vi "OSIPI OPCUA Server.vi"(11 "Main Queue Cluster":T65) -> ()   [LabVIEW 2018]
uses:
  support/Message Queue/Message Cluster.ctl
  <vilib>/OPCUA/controls/Supported Security Policies.ctl
  Drag and Drop/State Cluster.ctl
  Drag and Drop/Thumbnail Cluster.ctl
  Drag and Drop/Object Cluster.ctl
  <vilib>/Utility/miscctls.llb/LVRectTypeDef.ctl
  Drag and Drop/Object Type Enum.ctl
  <vilib>/Utility/miscctls.llb/LVPositionTypeDef.ctl
  Config Module/Controls/Main Config Cluster.ctl
  OPC Module Config.ctl
  Scale Module Folder/Measure Instrument/State Enum.ctl
  <vilib>/Utility/miscctls.llb/LVPoint32TypeDef.ctl
  OPC Settings.ctl
  Variable Data Cluster.ctl
  <vilib>/OPCUA/controls/NodeId.ctl
  <vilib>/OPCUA/controls/OPC UA StatusCode.ctl
  <vilib>/OPCUA/controls/Subscription ID.ctl
  <vilib>/OPCUA/controls/OPC UA Client Refnum.ctl
  <vilib>/OPCUA/controls/Subscription Data Change.ctl
  <vilib>/OPCUA/controls/Data Type.ctl
  Feed Module/Controls/Feed Module Config Cluster.ctl
  Feed Module/Controls/Feed Module Settings Cluster.ctl
  Ismatec ISM 831C/Controls/Ismatech Settings Cluster.ctl
  Masterflex 7550-30/Controls/Settings Cluster.ctl
  Mettler Toledo/Controls/Settings Cluster.ctl
  Bronkhorst M13 Flow Meter/Settings Cluster.ctl
  Measure Instrument/PID 2 Parameters Cluster.ctl
  Measure Instrument/PID Input Enum.ctl
  Measure Instrument/PID 2 Output Enum.ctl
  Tacmina QI/Tacmina QI DAQ Setting.ctl
  KNF Pump/Settings Cluster plus SIMDOS.ctl
  ASIA Pump/Pump Settings.ctl
  VICI M50 Party Mode/Settings Cluster.ctl
  FLOM Pump/Settings Cluster.ctl
  SSI PR Class/SSI PR Settings Cluster.ctl
  TT Module/Controls/TT Module Config Cluster.ctl
  Acquisition/Hardware Configuration.ctl
  Acquisition/Task Cluster.ctl
  PT Module/Controls/PT Module Config Cluster.ctl
  Scale Module Folder/Feed Module/Controls/Scale Module Config Cluster.ctl
  Scale Module Folder/Feed Module/Controls/Scale Module Settings Cluster.ctl
  Pump Module Folder/Pump Module Config Cluster.ctl
  Pump Module Folder/Pump Module Settings Cluster.ctl
  LabJack Module/Controls/U3 Module Config Cluster.ctl
  Decoration Module/Decoration Module Config Cluster.ctl
  Flow Module Folder/Feed Module/Controls/Flow Module Config Cluster.ctl
  Flow Module Folder/Feed Module/Controls/Flow Module Settings Cluster.ctl
  TCU Module/TCU Module Folder/TCU Module Config Cluster.ctl
  TCU Module/TCU Module Folder/TCU Module Settings Cluster.ctl
  TCU Module/TCU Module Folder/Measure Instrument/Output Devices.ctl
  Huber TCU/Huber Settings.ctl
  Lauda Integral XT-150 TCU/Lauda Settings.ctl
  Julabo Type 1 TCU/Julabo Type 1 TCU Folder/Julabo FP-50 Settings.ctl
  Huber Unistat 410 TCU/Huber Unistat 410 Settings.ctl
  Sequencing/Squence Control.ctl
  D-O Module Folder/D-O Module Config Cluster.ctl
  D-O Module Folder/Valve Clusters.ctl
  D-O Module Folder/D-O Module Settings Cluster.ctl
  D-O Module Folder/D-O Device Settings Cluster.ctl
  VICI Electronic Actuator/VICI Electronic Actuator Settings.ctl
  Pressure Regulator Control Module/Pressure Regulator/Controls/4-20mA Module Config Cluster.ctl
  Pressure Regulator Control Module/Pressure Regulator/Controls/4-20mA Module Settings Cluster.ctl
  Pressure Transmitter/Pressure Transmitter Device Settings.ctl
  Pressure Reg Module/Pressure Regulator Device Settings.ctl
  <vilib>/OPCUA/controls/OPC UA Variable Node Refnum.ctl
  <vilib>/OPCUA/controls/OPC UA Server Refnum.ctl
  Tag VIs/Tag FGV Operation Enum.ctl
  <vilib>/OPCUA/server/Write Double.vi
  <vilib>/OPCUA/NI OPC UA Server.lvlib
  support/Message Queue/Message Queue.lvlib
  Shared Variables/Dynamic Shared Variables.lvlib
  support/Message Queue/Enqueue Message (Single).vi
  TT Module/TT Module.lvlib
  Masterflex 7550-30/Masterflex 7550-30.lvlib
  Ismatec ISM 831C/Ismatec ISM 831C.lvlib
  Tacmina QI/Tacmina QI.lvlib
  KNF Pump/KNF SIMDOS.lvlib
  VICI M50 Party Mode/VICI M6 M50 Party Mode.lvlib
  FLOM Pump/FLOM Pump.lvlib
  ASIA Pump.lvlib
  Mettler Toledo/Mettler Toledo.lvlib
  Bronkhorst M13 Flow Meter/Bronkhorst M13 Flow Meter.lvlib
  SSI PR Class/SSI PR Pump.lvlib
  Feed Module/Feed Module.lvlib
  DAQ/DAQ.lvlib
  PT Module/PT Module.lvlib
  Scale Module Folder/Scale Module.lvlib
  Pump Module Folder/Pump Module.lvlib
  LabJack Module/U3 Module.lvlib
  Flow Module Folder/Flow Module.lvlib
  Huber TCU/Huber Ministat 230 TCU.lvlib
  Lauda Integral XT-150 TCU/Lauda TCU.lvlib
  Julabo Type 1 TCU/Julabo Type 1 TCU Folder/Julabo Type FP-50 TCU.lvlib
  Huber Unistat 410 TCU/Huber Unistat 410 TCU.lvlib
  TCU Module/TCU Module Folder/TCU Module.lvlib
  Sequencing/Sequencing Library.lvlib
  D-O Module Folder/D-O Module.lvlib
  Pressure Transmitter/Pressure Transmitter Library.lvlib
  Pressure Reg Module/Pressure Regulator Library.lvlib
  Pressure Regulator Control Module/Pressure Regulator/4-20mA Module.lvlib
  OPC UA.lvlib
  Scale Module Folder/Measure Instrument/Scale Module Engine.lvlib
  Config Module/Config Module.lvlib
  Drag and Drop/Drag and Drop.lvlib
  D-O Module Folder/DIO Valve/VICI Electronic Actuator.lvlib
panel:
  out "Array 3":T3(array[cluster])
  out "OPC UA server refnum out 3":T4
  out "Array 2":T5[](array[typedef]) items=["Good"=0, "Good_SubscriptionTransferred"=2949120, "Good_CompletesAsynchronously"=3014656, "Good_Overload"=3080192, "Good_Clamped"=3145728, "Good_LocalOverride"=9830400, "Good_EntryInserted"=10616832, "Good_EntryReplaced"=10682368, "Good_NoData"=10813440, "Good_MoreData"=10878976, "Good_CommunicationEvent"=10944512, "Good_ShutdownEvent"=11010048, "Good_CallAgain"=11075584, "Good_NonCriticalTimeout"=11141120, "Good_ResultsMayBeIncomplete"=12189696, "Good_DataIgnored"=14221312, "Uncertain"=1073741824, "Uncertain_ReferenceOutOfServer"=1080819712, "Uncertain_NoCommunicationLastUsableValue"=1083113472, "Uncertain_LastUsableValue"=1083179008, "Uncertain_SubstituteValue"=1083244544, "Uncertain_InitialValue"=1083310080, "Uncertain_SensorNotAccurate"=1083375616, "Uncertain_EngineeringUnitsExceeded"=1083441152, "Uncertain_SubNormal"=1083506688, "Uncertain_DataSubNormal"=1084489728, "Uncertain_ReferenceNotDeleted"=1086062592, "Uncertain_NotAllNodesAvailable"=1086324736, "Bad"=2147483648, "Bad_UnexpectedError"=2147549184, "Bad_InternalError"=2147614720, "Bad_OutOfMemory"=2147680256, "Bad_ResourceUnavailable"=2147745792, "Bad_CommunicationError"=2147811328, "Bad_EncodingError"=2147876864, "Bad_DecodingError"=2147942400, "Bad_EncodingLimitsExceeded"=2148007936, "Bad_UnknownResponse"=2148073472, "Bad_Timeout"=2148139008, "Bad_ServiceUnsupported"=2148204544, "Bad_Shutdown"=2148270080, "Bad_ServerNotConnected"=2148335616, "Bad_ServerHalted"=2148401152, "Bad_NothingToDo"=2148466688, "Bad_TooManyOperations"=2148532224, "Bad_DataTypeIdUnknown"=2148597760, "Bad_CertificateInvalid"=2148663296, "Bad_SecurityChecksFailed"=2148728832, "Bad_CertificateTimeInvalid"=2148794368, "Bad_CertificateIssuerTimeInvalid"=2148859904, "Bad_CertificateHostNameInvalid"=2148925440, "Bad_CertificateUriInvalid"=2148990976, "Bad_CertificateUseNotAllowed"=2149056512, "Bad_CertificateIssuerUseNotAllowed"=2149122048, "Bad_CertificateUntrusted"=2149187584, "Bad_CertificateRevocationUnknown"=2149253120, "Bad_CertificateIssuerRevocationUnknown"=2149318656, "Bad_CertificateRevoked"=2149384192, "Bad_CertificateIssuerRevoked"=2149449728, "Bad_UserAccessDenied"=2149515264, "Bad_IdentityTokenInvalid"=2149580800, "Bad_IdentityTokenRejected"=2149646336, "Bad_SecureChannelIdInvalid"=2149711872, "Bad_InvalidTimestamp"=2149777408, "Bad_NonceInvalid"=2149842944, "Bad_SessionIdInvalid"=2149908480, "Bad_SessionClosed"=2149974016, "Bad_SessionNotActivated"=2150039552, "Bad_SubscriptionIdInvalid"=2150105088, "Bad_RequestHeaderInvalid"=2150236160, "Bad_TimestampsToReturnInvalid"=2150301696, "Bad_RequestCancelledByClient"=2150367232, "Bad_NoCommunication"=2150694912, "Bad_WaitingForInitialData"=2150760448, "Bad_NodeIdInvalid"=2150825984, "Bad_NodeIdUnknown"=2150891520, "Bad_AttributeIdInvalid"=2150957056, "Bad_IndexRangeInvalid"=2151022592, "Bad_IndexRangeNoData"=2151088128, "Bad_DataEncodingInvalid"=2151153664, "Bad_DataEncodingUnsupported"=2151219200, "Bad_NotReadable"=2151284736, "Bad_NotWritable"=2151350272, "Bad_OutOfRange"=2151415808, "Bad_NotSupported"=2151481344, "Bad_NotFound"=2151546880, "Bad_ObjectDeleted"=2151612416, "Bad_NotImplemented"=2151677952, "Bad_MonitoringModeInvalid"=2151743488, "Bad_MonitoredItemIdInvalid"=2151809024, "Bad_MonitoredItemFilterInvalid"=2151874560, "Bad_MonitoredItemFilterUnsupported"=2151940096, "Bad_FilterNotAllowed"=2152005632, "Bad_StructureMissing"=2152071168, "Bad_EventFilterInvalid"=2152136704, "Bad_ContentFilterInvalid"=2152202240, "Bad_FilterOperandInvalid"=2152267776, "Bad_ContinuationPointInvalid"=2152333312, "Bad_NoContinuationPoints"=2152398848, "Bad_ReferenceTypeIdInvalid"=2152464384, "Bad_BrowseDirectionInvalid"=2152529920, "Bad_NodeNotInView"=2152595456, "Bad_ServerUriInvalid"=2152660992, "Bad_ServerNameMissing"=2152726528, "Bad_DiscoveryUrlMissing"=2152792064, "Bad_SempahoreFileMissing"=2152857600, "Bad_RequestTypeInvalid"=2152923136, "Bad_SecurityModeRejected"=2152988672, "Bad_SecurityPolicyRejected"=2153054208, "Bad_TooManySessions"=2153119744, "Bad_UserSignatureInvalid"=2153185280, "Bad_ApplicationSignatureInvalid"=2153250816, "Bad_NoValidCertificates"=2153316352, "Bad_RequestCancelledByRequest"=2153381888, "Bad_ParentNodeIdInvalid"=2153447424, "Bad_ReferenceNotAllowed"=2153512960, "Bad_NodeIdRejected"=2153578496, "Bad_NodeIdExists"=2153644032, "Bad_NodeClassInvalid"=2153709568, "Bad_BrowseNameInvalid"=2153775104, "Bad_BrowseNameDuplicated"=2153840640, "Bad_NodeAttributesInvalid"=2153906176, "Bad_TypeDefinitionInvalid"=2153971712, "Bad_SourceNodeIdInvalid"=2154037248, "Bad_TargetNodeIdInvalid"=2154102784, "Bad_DuplicateReferenceNotAllowed"=2154168320, "Bad_InvalidSelfReference"=2154233856, "Bad_ReferenceLocalOnly"=2154299392, "Bad_NoDeleteRights"=2154364928, "Bad_ServerIndexInvalid"=2154430464, "Bad_ViewIdUnknown"=2154496000, "Bad_TooManyMatches"=2154627072, "Bad_QueryTooComplex"=2154692608, "Bad_NoMatch"=2154758144, "Bad_MaxAgeInvalid"=2154823680, "Bad_HistoryOperationInvalid"=2154889216, "Bad_HistoryOperationUnsupported"=2154954752, "Bad_WriteNotSupported"=2155020288, "Bad_TypeMismatch"=2155085824, "Bad_MethodInvalid"=2155151360, "Bad_ArgumentsMissing"=2155216896, "Bad_TooManySubscriptions"=2155282432, "Bad_TooManyPublishRequests"=2155347968, "Bad_NoSubscription"=2155413504, "Bad_SequenceNumberUnknown"=2155479040, "Bad_MessageNotAvailable"=2155544576, "Bad_InsufficientClientProfile"=2155610112, "Bad_TcpServerTooBusy"=2155675648, "Bad_TcpMessageTypeInvalid"=2155741184, "Bad_TcpSecureChannelUnknown"=2155806720, "Bad_TcpMessageTooLarge"=2155872256, "Bad_TcpNotEnoughResources"=2155937792, "Bad_TcpInternalError"=2156003328, "Bad_TcpEndpointUrlInvalid"=2156068864, "Bad_RequestInterrupted"=2156134400, "Bad_RequestTimeout"=2156199936, "Bad_SecureChannelClosed"=2156265472, "Bad_SecureChannelTokenUnknown"=2156331008, "Bad_SequenceNumberInvalid"=2156396544, "Bad_ConfigurationError"=2156462080, "Bad_NotConnected"=2156527616, "Bad_DeviceFailure"=2156593152, "Bad_SensorFailure"=2156658688, "Bad_OutOfService"=2156724224, "Bad_DeadbandFilterInvalid"=2156789760, "Bad_RefreshInProgress"=2157379584, "Bad_ConditionAlreadyDisabled"=2157445120, "Bad_ConditionDisabled"=2157510656, "Bad_EventIdUnknown"=2157576192, "Bad_NoData"=2157641728, "Bad_DataLost"=2157772800, "Bad_DataUnavailable"=2157838336, "Bad_EntryExists"=2157903872, "Bad_NoEntryExists"=2157969408, "Bad_TimestampNotSupported"=2158034944, "Bad_InvalidArgument"=2158690304, "Bad_ConnectionRejected"=2158755840, "Bad_Disconnect"=2158821376, "Bad_ConnectionClosed"=2158886912, "Bad_InvalidState"=2158952448, "Bad_EndOfStream"=2159017984, "Bad_NoDataAvailable"=2159083520, "Bad_WaitingForResponse"=2159149056, "Bad_OperationAbandoned"=2159214592, "Bad_ExpectedStreamToBlock"=2159280128, "Bad_WouldBlock"=2159345664, "Bad_SyntaxError"=2159411200, "Bad_MaxConnectionsReached"=2159476736, "Bad_RequestTooLarge"=2159542272, "Bad_ResponseTooLarge"=2159607808, "Bad_EventNotAcknowledgeable"=2159738880, "Bad_InvalidTimestampArgument"=2159869952, "Bad_ProtocolVersionUnsupported"=2159935488, "Bad_StateNotActive"=2160001024, "Bad_FilterOperatorInvalid"=2160132096, "Bad_FilterOperatorUnsupported"=2160197632, "Bad_FilterOperandCountMismatch"=2160263168, "Bad_FilterElementInvalid"=2160328704, "Bad_FilterLiteralInvalid"=2160394240, "Bad_IdentityChangeNotSupported"=2160459776, "Bad_NotTypeDefinition"=2160590848, "Bad_ViewTimestampInvalid"=2160656384, "Bad_ViewParameterMismatch"=2160721920, "Bad_ViewVersionInvalid"=2160787456, "Bad_ConditionAlreadyEnabled"=2160852992, "Bad_DialogNotActive"=2160918528, "Bad_DialogResponseInvalid"=2160984064, "Bad_ConditionBranchAlreadyAcked"=2161049600, "Bad_ConditionBranchAlreadyConfirmed"=2161115136, "Bad_ConditionAlreadyShelved"=2161180672, "Bad_ConditionNotShelved"=2161246208, "Bad_ShelvingTimeOutOfRange"=2161311744, "Bad_AggregateListMismatch"=2161377280, "Bad_AggregateNotSupported"=2161442816, "Bad_AggregateInvalidInputs"=2161508352, "Bad_BoundNotFound"=2161573888, "Bad_BoundNotSupported"=2161639424, "Bad_AggregateConfigurationRejected"=2161770496, "Bad_TooManyMonitoredItems"=2161836032]
  out "OPC UA server refnum out":T4
  out "Array":T3(array[cluster])
  in  "?":T6={"VI refs"=[], "Queues"=[], "[Thumbnails]"=[], "Drag Object Idx"=0, "[Objects]"=[], "Active Object"=0, "Drop Offset"={"Left"=0, "Top"=0}, "Process Name"="", "Main Config"={"OPC Module Configs"=[], "Feed Module Configs"=[], "Log File Path"=path "", "TT Module Configs"=[], "DAQ Config"={"Tasks"=[]}, "PT Module Configs"=[], "Scale Module Configs"=[], "Pump Module Configs"=[], "U3 Module Configs"=[{"GUID"="", "Drop Coords"={"Horizontal"=0, "Vertical"=0}, "AI Channel Number"=enum."Default", "Process Name"="", "Input Channel Numeric Alarm Settings"=[]}], "Decoration Module Configs"=[], "Flow Module Configs"=[], "TCU Module Configs"=[], "Steps"=[], "DO Module Configs"=[], "PR Module Configs"=[], "Cycle Period"=0.0}, "Campaign Filepath"=path "", "Config Changed?"=FALSE} {"Main Config"."PR Module Configs"."Settings"."PID 2 Parameters"."output range"."output low" format="%.2f"; "Main Config"."PR Module Configs"."Settings"."PID 2 Parameters"."output range"."output high" min=0.0 max=100.0 format="%.2f"; "Main Config"."PR Module Configs"."Settings"."PID 2 Parameters"."PID gains"."derivative time (Td, min)" format="%.3f"; "Main Config"."PR Module Configs"."Settings"."PID 2 Parameters"."PID gains"."integral time (Ti, min)" format="%.3f"; "Main Config"."PR Module Configs"."Settings"."PID 2 Parameters"."PID gains"."proportional gain (Kc)" format="%.3f"; "Main Config"."Steps"."Control" items=["Pump %", "Setpoint"]; "Main Config"."TCU Module Configs"."Settings"."Julabo FP-50 Settings"."Pump Power" min=0 max=8 step=1; "Main Config"."TCU Module Configs"."Settings"."Lauda Settings"."Pump Power" min=0 max=8 step=1; "Main Config"."Pump Module Configs"."Settings"."ASIA Pump C"."channel" min=0 max=1 step=1; "Main Config"."Pump Module Configs"."Settings"."Masterflex"."Pump Number" min=1.0 max=20.0 step=1.0; "Main Config"."Pump Module Configs"."Settings"."Ismatech"."Pump Number" min=1.0 max=20.0 step=1.0; "Main Config"."Feed Module Configs"."Settings"."output range"."output low" min=0.0 max=100.0 format="%.2f"; "Main Config"."Feed Module Configs"."Settings"."output range"."output high" format="%.2f"; "Main Config"."Feed Module Configs"."Settings"."PID 2 Parameters"."PID gains"."derivative time (Td, min)" format="%.3f"; "Main Config"."Feed Module Configs"."Settings"."PID 2 Parameters"."PID gains"."integral time (Ti, min)" format="%.3f"; "Main Config"."Feed Module Configs"."Settings"."PID 2 Parameters"."PID gains"."proportional gain (Kc)" format="%.3f"; "Main Config"."Feed Module Configs"."Settings"."ASIA Pump C"."channel" min=0 max=1 step=1; "Main Config"."Feed Module Configs"."Settings"."Ismatech"."Pump Number" min=1.0 max=20.0 step=1.0; "Main Config"."Feed Module Configs"."Settings"."Masterflex"."Pump Number" min=1.0 max=20.0 step=1.0}
  out "Tag Values":dbl[](array[numeric])
  out "Tag Names":string[](array[string])
  in  "?":T6 {"Main Config"."PR Module Configs"."Settings"."PID 2 Parameters"."output range"."output low" format="%.2f"; "Main Config"."PR Module Configs"."Settings"."PID 2 Parameters"."output range"."output high" min=0.0 max=100.0 format="%.2f"; "Main Config"."PR Module Configs"."Settings"."PID 2 Parameters"."PID gains"."derivative time (Td, min)" format="%.3f"; "Main Config"."PR Module Configs"."Settings"."PID 2 Parameters"."PID gains"."integral time (Ti, min)" format="%.3f"; "Main Config"."PR Module Configs"."Settings"."PID 2 Parameters"."PID gains"."proportional gain (Kc)" format="%.3f"; "Main Config"."Steps"."Control" items=["Pump %", "Setpoint"]; "Main Config"."TCU Module Configs"."Settings"."Julabo FP-50 Settings"."Pump Power" min=0 max=8 step=1; "Main Config"."TCU Module Configs"."Settings"."Lauda Settings"."Pump Power" min=0 max=8 step=1; "Main Config"."Pump Module Configs"."Settings"."ASIA Pump C"."channel" min=0 max=1 step=1; "Main Config"."Pump Module Configs"."Settings"."Masterflex"."Pump Number" min=1.0 max=20.0 step=1.0; "Main Config"."Pump Module Configs"."Settings"."Ismatech"."Pump Number" min=1.0 max=20.0 step=1.0; "Main Config"."Feed Module Configs"."Settings"."output range"."output low" min=0.0 max=100.0 format="%.2f"; "Main Config"."Feed Module Configs"."Settings"."output range"."output high" format="%.2f"; "Main Config"."Feed Module Configs"."Settings"."PID 2 Parameters"."PID gains"."derivative time (Td, min)" format="%.3f"; "Main Config"."Feed Module Configs"."Settings"."PID 2 Parameters"."PID gains"."integral time (Ti, min)" format="%.3f"; "Main Config"."Feed Module Configs"."Settings"."PID 2 Parameters"."PID gains"."proportional gain (Kc)" format="%.3f"; "Main Config"."Feed Module Configs"."Settings"."ASIA Pump C"."channel" min=0 max=1 step=1; "Main Config"."Feed Module Configs"."Settings"."Ismatech"."Pump Number" min=1.0 max=20.0 step=1.0; "Main Config"."Feed Module Configs"."Settings"."Masterflex"."Pump Number" min=1.0 max=20.0 step=1.0}
  in  "supported security policies (None)":T64={"None"=TRUE, "Sign with Basic128Rsa15"=TRUE, "Sign and Encrypt with Basic128Rsa15"=TRUE, "Sign with Basic256"=TRUE, "Sign and Encrypt with Basic256"=TRUE}
  out "server endpoint URL":string
  # "Instrument Settings"
  # "Instrument Settings"
  # "Output Instruments"
  # "Flow Meter Settings"
  # "Output Instruments"
  # "Scale Settings"
  # "Output Instruments"
  # "Input Instruments"
  # "Instrument Settings"
  # "Instrument Settings"
  # "Output Instruments"
  # "Flow Meter Settings"
  # "Output Instruments"
  # "Scale Settings"
  # "Output Instruments"
  # "Input Instruments"
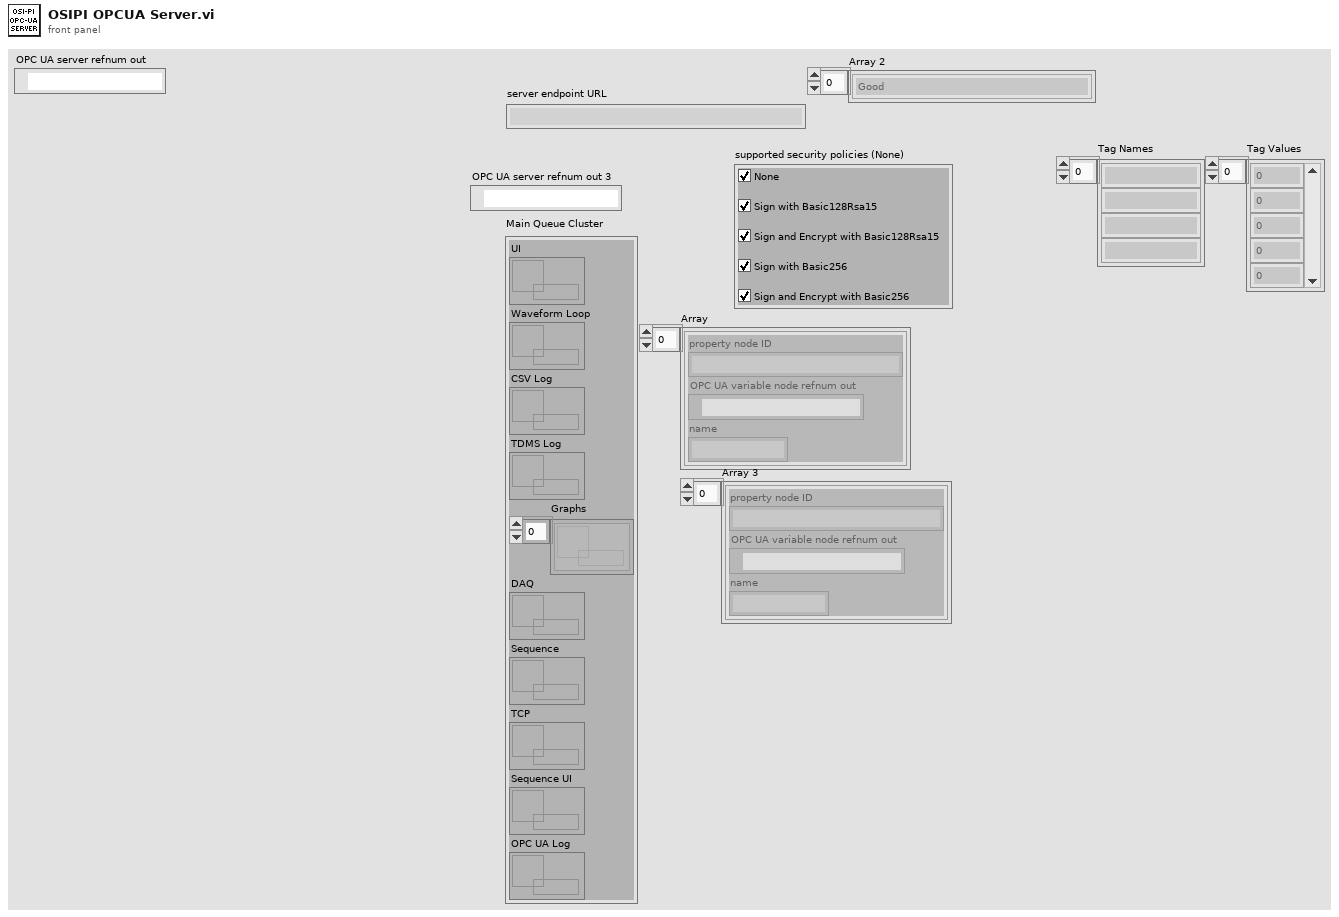
[diagram p1: front panel]
types:
  T1 = typedef "NodeId.ctl" = string
  T2 = typedef "OPC UA Variable Node Refnum.ctl" = refnum<k21>
  T3 = cluster{"property node ID":T1, "OPC UA variable node refnum out":T2, "name":string}[]
  T4 = typedef "OPC UA Server Refnum.ctl" = refnum<k21>
  T5 = typedef "OPC UA StatusCode.ctl" = u32
  T6 = typedef "Drag and Drop.lvlib/State Cluster.ctl" = cluster{"VI refs":refnum<vi>[], "Queues":refnum<queue>[], "[Thumbnails]":T7[], "Drag Object Idx":i32, "[Objects]":T8[], "Active Object":i32, "Drop Offset":T11, "Process Name":string, "Main Config":T12, "Campaign Filepath":path, "Config Changed?":bool}
  T7 = typedef "Thumbnail Cluster.ctl" = cluster{"Path":path, "Rectangle":cluster{"left":i16, "top":i16, "right":i16, "bottom":i16}}
  T8 = typedef "Object Cluster.ctl" = cluster{"BMP Path":path, "Anchor Position":cluster{"X":i32, "Y":i32}, "Hot Spot":T9, "Type":T10, "Parameters":variant}
  T9 = typedef "LVRectTypeDef.ctl" = cluster{"Left":i16, "Top":i16, "Right":i16, "Bottom":i16}
  T10 = typedef "Object Type Enum.ctl" = enum16{"Icon", "Line", "Text", "Feed Module"}
  T11 = typedef "LVPositionTypeDef.ctl" = cluster{"Left":i32, "Top":i32}
  T12 = typedef "Config Module.lvlib/Main Config Cluster.ctl" = cluster{"OPC Module Configs":T13[], "Feed Module Configs":T20[], "Log File Path":path, "TT Module Configs":T35[], "DAQ Config":T36, "PT Module Configs":T38[], "Scale Module Configs":T39[], "Pump Module Configs":T41[], "U3 Module Configs":T43[], "Decoration Module Configs":T44[], "Flow Module Configs":T45[], "TCU Module Configs":T47[], "Steps":T54[], "DO Module Configs":T55[], "PR Module Configs":T60[], "Cycle Period":dbl}
  T13 = typedef "OPC UA.lvlib/OPC Module Config.ctl" = cluster{"State":T14, "GUID":string, "Drop Coords":T15, "Configuration":T16, "First Iteration":bool, "Data":cluster{"Object Name":string, "Variable Array":T17[]}[], "Process Name":string, "Load Count":i32, "Log Started":bool, "subscription ID out":T18, "OPC UA client refnum out":T19, "Event Registration Refnum":refnum<event-registration>, "Start Time":timestamp, "Current Time":timestamp}
  T14 = typedef "Scale Module.lvlib/Scale Module Engine.lvlib/State Enum.ctl" = enum16{"Measuring", "Idle"}
  T15 = typedef "LVPoint32TypeDef.ctl" = cluster{"Horizontal":i32, "Vertical":i32}
  T16 = typedef "OPC UA.lvlib/OPC Settings.ctl" = cluster{"Cycle Period":dbl, "server endpoint URL":string, "security policy":cluster{"message mode":enum16{"None", "Sign", "Sign and Encrypt"}, "security":enum16{"Basic256", "Basic128Rsa15"}}, "Trust Any Server":bool}
  T17 = typedef "OPC UA.lvlib/Variable Data Cluster.ctl" = cluster{"node ID":T1, "browse name":string, "status":T5, "timestamp":timestamp, "value ":variant}
  T18 = typedef "Subscription ID.ctl" = u32
  T19 = typedef "OPC UA Client Refnum.ctl" = refnum<k21>
  T20 = typedef "Feed Module.lvlib/Feed Module Config Cluster.ctl" = cluster{"GUID":string, "Drop Coords":T15, "Process Name":string, "Settings":T21, "Settings Load Count":i32, "OP Load Count":i32}
  T21 = typedef "Feed Module.lvlib/Feed Module Settings Cluster.ctl" = cluster{"Cycle Period":dbl, "Ismatech":T22, "Masterflex":T23, "Mettler":T24, "Bronkhorst M13 Flow Meter":T25, "PID 2 Parameters":T26, "Manual Entry":dbl, "Auto?":bool, "output range":cluster{"output high":dbl, "output low":dbl}, "Bronkhorst M14":T24, "Tacmina Settings":T29, "KNF SIMDOS Settings":T30, "ASIA Pump C":T31, "VICI Settings":T32, "FLOM Settings":T33, "SSI PR Settings":T34}
  T22 = typedef "Ismatec ISM 831C.lvlib/Ismatech Settings Cluster.ctl" = cluster{"VISA resource name":refnum<visa-resource-name>, "Simulated?":bool, "Pump Number":dbl, "Reverse?":bool}
  T23 = typedef "Masterflex 7550-30.lvlib/Settings Cluster.ctl" = cluster{"VISA resource name":refnum<visa-resource-name>, "Simulated?":bool, "Pump Number":dbl, "Reverse?":bool}
  T24 = typedef "Mettler Toledo.lvlib/Settings Cluster.ctl" = cluster{"VISA resource name":refnum<visa-resource-name>, "Simulated?":bool}
  T25 = typedef "Bronkhorst M13 Flow Meter.lvlib/Settings Cluster.ctl" = cluster{"VISA resource name":refnum<visa-resource-name>, "Simulated?":bool}
  T26 = typedef "PID 2 Parameters Cluster.ctl" = cluster{"Input Device":T27, "Output Device":T28, "Setpoint":dbl, "PID gains":cluster{"proportional gain (Kc)":dbl, "integral time (Ti, min)":dbl, "derivative time (Td, min)":dbl}}
  T27 = typedef "PID Input Enum.ctl" = enum16{"Default", "Bronkhorst M13", "Bronkhorst M14", "Scale Rate of Change"}
  T28 = typedef "PID 2 Output Enum.ctl" = enum16{"Default", "Ismatec ISM 831C", "Masterflex 7550-30", "VICI", "Tacmina QI", "KNF SIMDOS", "ASIA Type C", "FLOM UI-22-11", "SSI PR"}
  T29 = typedef "Tacmina QI.lvlib/Tacmina QI DAQ Setting.ctl" = cluster{"Analog DAQ Task":refnum<k21>, "Digital DAQ Task":refnum<k21>}
  T30 = typedef "KNF SIMDOS.lvlib/Settings Cluster plus SIMDOS.ctl" = cluster{"VISA resource name":refnum<visa-resource-name>, "Simulated?":bool}
  T31 = typedef "ASIA Pump.lvlib/Pump Settings.ctl" = cluster{"ASIA Pump #":i32, "channel":i32, "Simulated":bool}
  T32 = typedef "VICI M6 M50 Party Mode.lvlib/Settings Cluster.ctl" = cluster{"VISA resource name":refnum<visa-resource-name>, "Simulated?":bool, "Pump Letter":string, "Reverse?":bool}
  T33 = typedef "FLOM Pump.lvlib/Settings Cluster.ctl" = cluster{"VISA resource name":refnum<visa-resource-name>, "Simulated?":bool, "Pump Number":dbl}
  T34 = typedef "SSI PR Pump.lvlib/SSI PR Settings Cluster.ctl" = cluster{"VISA resource name":refnum<visa-resource-name>, "Simulated?":bool}
  T35 = typedef "TT Module.lvlib/TT Module Config Cluster.ctl" = cluster{"GUID":string, "Drop Coords":T15, "Input Channel Tag Name ":string, "Process Name":string, "Input Channel Numeric Alarm Settings":cluster{"enable? (F)":bool, "name":string, "alarm type":enum16{"HI_HI", "HI", "LO", "LO_LO"}, "level/change":dbl, "deadband/time":dbl, "priority":u32, "ack type":enum16{"Auto", "User", "None", "Each Occurrence"}, "area":string, "description":string, "log? (T)":bool}[]}
  T36 = typedef "DAQ.lvlib/Hardware Configuration.ctl" = cluster{"Tasks":T37[]}
  T37 = typedef "Task Cluster.ctl" = cluster{"DAQmx Task":refnum<k21>, "Read-Write Radio":enum32{"Read", "Write"}}
  T38 = typedef "PT Module.lvlib/PT Module Config Cluster.ctl" = cluster{"GUID":string, "Drop Coords":T15, "Input Channel Tag Name ":string, "Process Name":string, "Input Channel Numeric Alarm Settings":cluster{"enable? (F)":bool, "name":string, "alarm type":enum16{"HI_HI", "HI", "LO", "LO_LO"}, "level/change":dbl, "deadband/time":dbl, "priority":u32, "ack type":enum16{"Auto", "User", "None", "Each Occurrence"}, "area":string, "description":string, "log? (T)":bool}[]}
  T39 = typedef "Scale Module.lvlib/Scale Module Config Cluster.ctl" = cluster{"GUID":string, "Drop Coords":T15, "Process Name":string, "Settings":T40, "Load Count":i32}
  T40 = typedef "Scale Module.lvlib/Scale Module Settings Cluster.ctl" = cluster{"Cycle Period":dbl, "Mettler":T24, "Scale Type":string}
  T41 = typedef "Pump Module.lvlib/Pump Module Config Cluster.ctl" = cluster{"GUID":string, "Drop Coords":T15, "Process Name":string, "Settings":T42, "Load Count":i32}
  T42 = typedef "Pump Module.lvlib/Pump Module Settings Cluster.ctl" = cluster{"Cycle Period":dbl, "Ismatech":T22, "Masterflex":T23, "Manual Entry":dbl, "VICI Settings":T32, "Output Device":T28, "Tacmina Settings":T29, "KNF SIMDOS Settings":T30, "ASIA Pump C":T31, "FLOM Settings":T33, "Pump Calibration File":path, "Calibration":dbl, "Pump Cal Enum":u16, "SSI PR Settings":T34}
  T43 = typedef "U3 Module.lvlib/U3 Module Config Cluster.ctl" = cluster{"GUID":string, "Drop Coords":T15, "AI Channel Number":enum16{"Default", "AI0", "AI1", "AI2", "AI3", "AI4", "AI5", "AI6", "AI7"}, "Process Name":string, "Input Channel Numeric Alarm Settings":cluster{"enable? (F)":bool, "name":string, "alarm type":enum16{"HI_HI", "HI", "LO", "LO_LO"}, "level/change":dbl, "deadband/time":dbl, "priority":u32, "ack type":enum16{"Auto", "User", "None", "Each Occurrence"}, "area":string, "description":string, "log? (T)":bool}[]}
  T44 = typedef "Decoration Module Config Cluster.ctl" = cluster{"GUID":string, "Drop Coords":T15, "Decoration Filepath":path}
  T45 = typedef "Flow Module.lvlib/Flow Module Config Cluster.ctl" = cluster{"GUID":string, "Drop Coords":T15, "Process Name":string, "Settings":T46, "Load Count":i32}
  T46 = typedef "Flow Module.lvlib/Flow Module Settings Cluster.ctl" = cluster{"Cycle Period":dbl, "Bronkhorst M13":T24, "Flow Meter Type":string, "Bronkhorst M14":T24}
  T47 = typedef "TCU Module.lvlib/TCU Module Config Cluster.ctl" = cluster{"GUID":string, "Drop Coords":T15, "Process Name":string, "Settings":T48, "Load Count":i32, "Power Level Changed":bool}
  T48 = typedef "TCU Module.lvlib/TCU Module Settings Cluster.ctl" = cluster{"Cycle Period":dbl, "Setpoint Entry":dbl, "Output Device":T49, "Huber Ministat 230 Settings":T50, "Lauda Settings":T51, "Julabo FP-50 Settings":T52, "Internal Control?":bool, "Huber Unistat 410 Settings":T53}
  T49 = typedef "Output Devices.ctl" = enum16{"Default", "Huber Ministat 230", "Huber Unistat 410", "Lauda XT-150", "Julabo FP-50"}
  T50 = typedef "Huber Ministat 230 TCU.lvlib/Huber Settings.ctl" = cluster{"VISA resource name":refnum<visa-resource-name>, "Simulated?":bool}
  T51 = typedef "Lauda TCU.lvlib/Lauda Settings.ctl" = cluster{"VISA resource name":refnum<visa-resource-name>, "Simulated?":bool, "Pump Power":i32}
  T52 = typedef "Julabo Type FP-50 TCU.lvlib/Julabo FP-50 Settings.ctl" = cluster{"VISA resource name":refnum<visa-resource-name>, "Simulated?":bool, "Pump Power":i32}
  T53 = typedef "Huber Unistat 410 TCU.lvlib/Huber Unistat 410 Settings.ctl" = cluster{"VISA resource name":refnum<visa-resource-name>, "Simulated?":bool}
  T54 = typedef "Sequencing Library.lvlib/Squence Control.ctl" = cluster{"Module":string, "Control":u16, "Value":dbl, "Wait (sec)":dbl}
  T55 = typedef "D-O Module.lvlib/D-O Module Config Cluster.ctl" = cluster{"GUID":string, "Drop Coords":T15, "Process Name":string, "Settings":T56, "Load Count":i32}
  T56 = typedef "D-O Module.lvlib/Valve Clusters.ctl" = cluster{"Valve Settings":T57, "Valve Type":enum16{"Digital Output Valve", "VICI Electronic Actuator"}, "Time On (Sec)":dbl, "Time Off (Sec)":dbl}
  T57 = typedef "D-O Module.lvlib/D-O Module Settings Cluster.ctl" = cluster{"D-O Settings":T58, "VICI Electronic Actuator":T59}
  T58 = typedef "D-O Module.lvlib/D-O Device Settings Cluster.ctl" = cluster{"DAQmx Task Name":refnum<k21>, "Output Channel":u16, "Output Channel Names":string[], "Run?":bool}
  T59 = typedef "VICI Electronic Actuator.lvlib/VICI Electronic Actuator Settings.ctl" = cluster{"VISA resource name":refnum<visa-resource-name>, "Mode":enum16{"Two Positions With Stops", "Two Positions Without Stops", "Mutiposition"}, "Simulated":bool}
  T60 = typedef "4-20mA Module.lvlib/4-20mA Module Config Cluster.ctl" = cluster{"GUID":string, "Drop Coords":T15, "Process Name":string, "Settings":T61, "Settings Load Count":i32}
  T61 = typedef "4-20mA Module.lvlib/4-20mA Module Settings Cluster.ctl" = cluster{"Cycle Period":dbl, "PID 2 Parameters":cluster{"Input Device":enum16{"Default", "4-20mA"}, "Output Device":enum16{"Default", "Equilibar Pressure Reg", "Flow Regulator"}, "Setpoint":dbl, "PID gains":cluster{"proportional gain (Kc)":dbl, "integral time (Ti, min)":dbl, "derivative time (Td, min)":dbl}, "output range":cluster{"output low":dbl, "output high":dbl}}, "Manual Entry":dbl, "Auto?":bool, "4-20mA Input Settings":T62, "4-20mA Out Settings":T63, "Input Channel Tag Name ":string}
  T62 = typedef "Pressure Transmitter Library.lvlib/Pressure Transmitter Device Settings.ctl" = cluster{"Input Channel ":u16}
  T63 = typedef "Pressure Regulator Library.lvlib/Pressure Regulator Device Settings.ctl" = cluster{"Output DAQ Task":refnum<k21>}
  T64 = typedef "Supported Security Policies.ctl" = cluster{"None":bool, "Sign with Basic128Rsa15":bool, "Sign and Encrypt with Basic128Rsa15":bool, "Sign with Basic256":bool, "Sign and Encrypt with Basic256":bool}
  T65 = cluster{"UI":refnum<queue>, "Waveform Loop":refnum<queue>, "CSV Log":refnum<queue>, "TDMS Log":refnum<queue>, "Graphs":refnum<queue>[], "DAQ":refnum<queue>, "Sequence":refnum<queue>, "TCP":refnum<queue>, "Sequence UI":refnum<queue>, "OPC UA Log":refnum<queue>}
  T66 = typedef "Data Type.ctl" = u16
  T67 = cluster{"name":string, "data type":T66, "access level":u16, "description":string}
  T68 = cluster{"property node ID":T1, "OPC UA variable node refnum out":T2, "name":string}
  T69 = typedef "Tag FGV Operation Enum.ctl" = enum16{"Init", "Set Notification Queue", "Create Tag", "Commit", "Write Tag (Numeric)", "Write Tag (Boolean)", "Read All Tags", "Read One Tag", "Delete Tag Category", "Set Alarm Parameters (Numeric)", "Set Alarm Parameters (Boolean)", "Enable All Alarms", "Disable All Alarms", "Delete All Tags", "Read Alarms", "Ack Alarm"}
  T70 = typedef "Feed Module.lvlib/Feed Module Tag Names Cluster.ctl" = cluster{"Pump Flow Tag":string, "PID 2 Out Tag":string, "Scale Tag":string, "Density Tag":string, "FL Temp":string, "Input Device Tag":string, "Output Device Tag":string, "Pump's Flow":string, "Pump's Pressure":string, "Overpressure Tag":string}
  T71 = typedef "Pump Module.lvlib/Pump Module Tag Names Cluster.ctl" = cluster{"Pump Speed":string, "Pump Flow":string, "Pump Pressure":string, "Output Device Tag":string, "Overpressure Tag":string}
  T72 = typedef "Flow Module.lvlib/Tag Cluster.ctl" = cluster{"Flow Tag":string, "Input Disconnected":string, "Density Tag":string, "Temp Tag":string}
  T73 = typedef "TCU Module.lvlib/TCU Module Tag Names Cluster.ctl" = cluster{"TCU Temp":string, "Output Device Tag":string, "TCU Speed":string}
  T74 = typedef "4-20mA Module.lvlib/4-20mA Module Tag Names Cluster.ctl" = cluster{"4-20mA Input":string, "PID 2 Out Tag":string, "4-20mA Output":string, "Input Device Tag":string, "Output Device Tag":string}
  T75 = cluster{"Feed Module Tags Array":T70[], "DAQ Tags Array":string[], "Scale Tags Array":cluster{"Scale Value":string, "Scale Error":string}[], "Pump Module Tags Array":T71[], "Flow Module Tags Array":T72[], "TCU Module Tags Array":T73[], "PR Module Tags Array":T74[], "OPC Module Tags Array":cluster{"OPC UA Error":string, "Array of Names":string[]}[]}
  T76 = cluster{"Scale Value":string, "Scale Error":string}[]
  T77 = cluster{"OPC UA Error":string, "Array of Names":string[]}[]
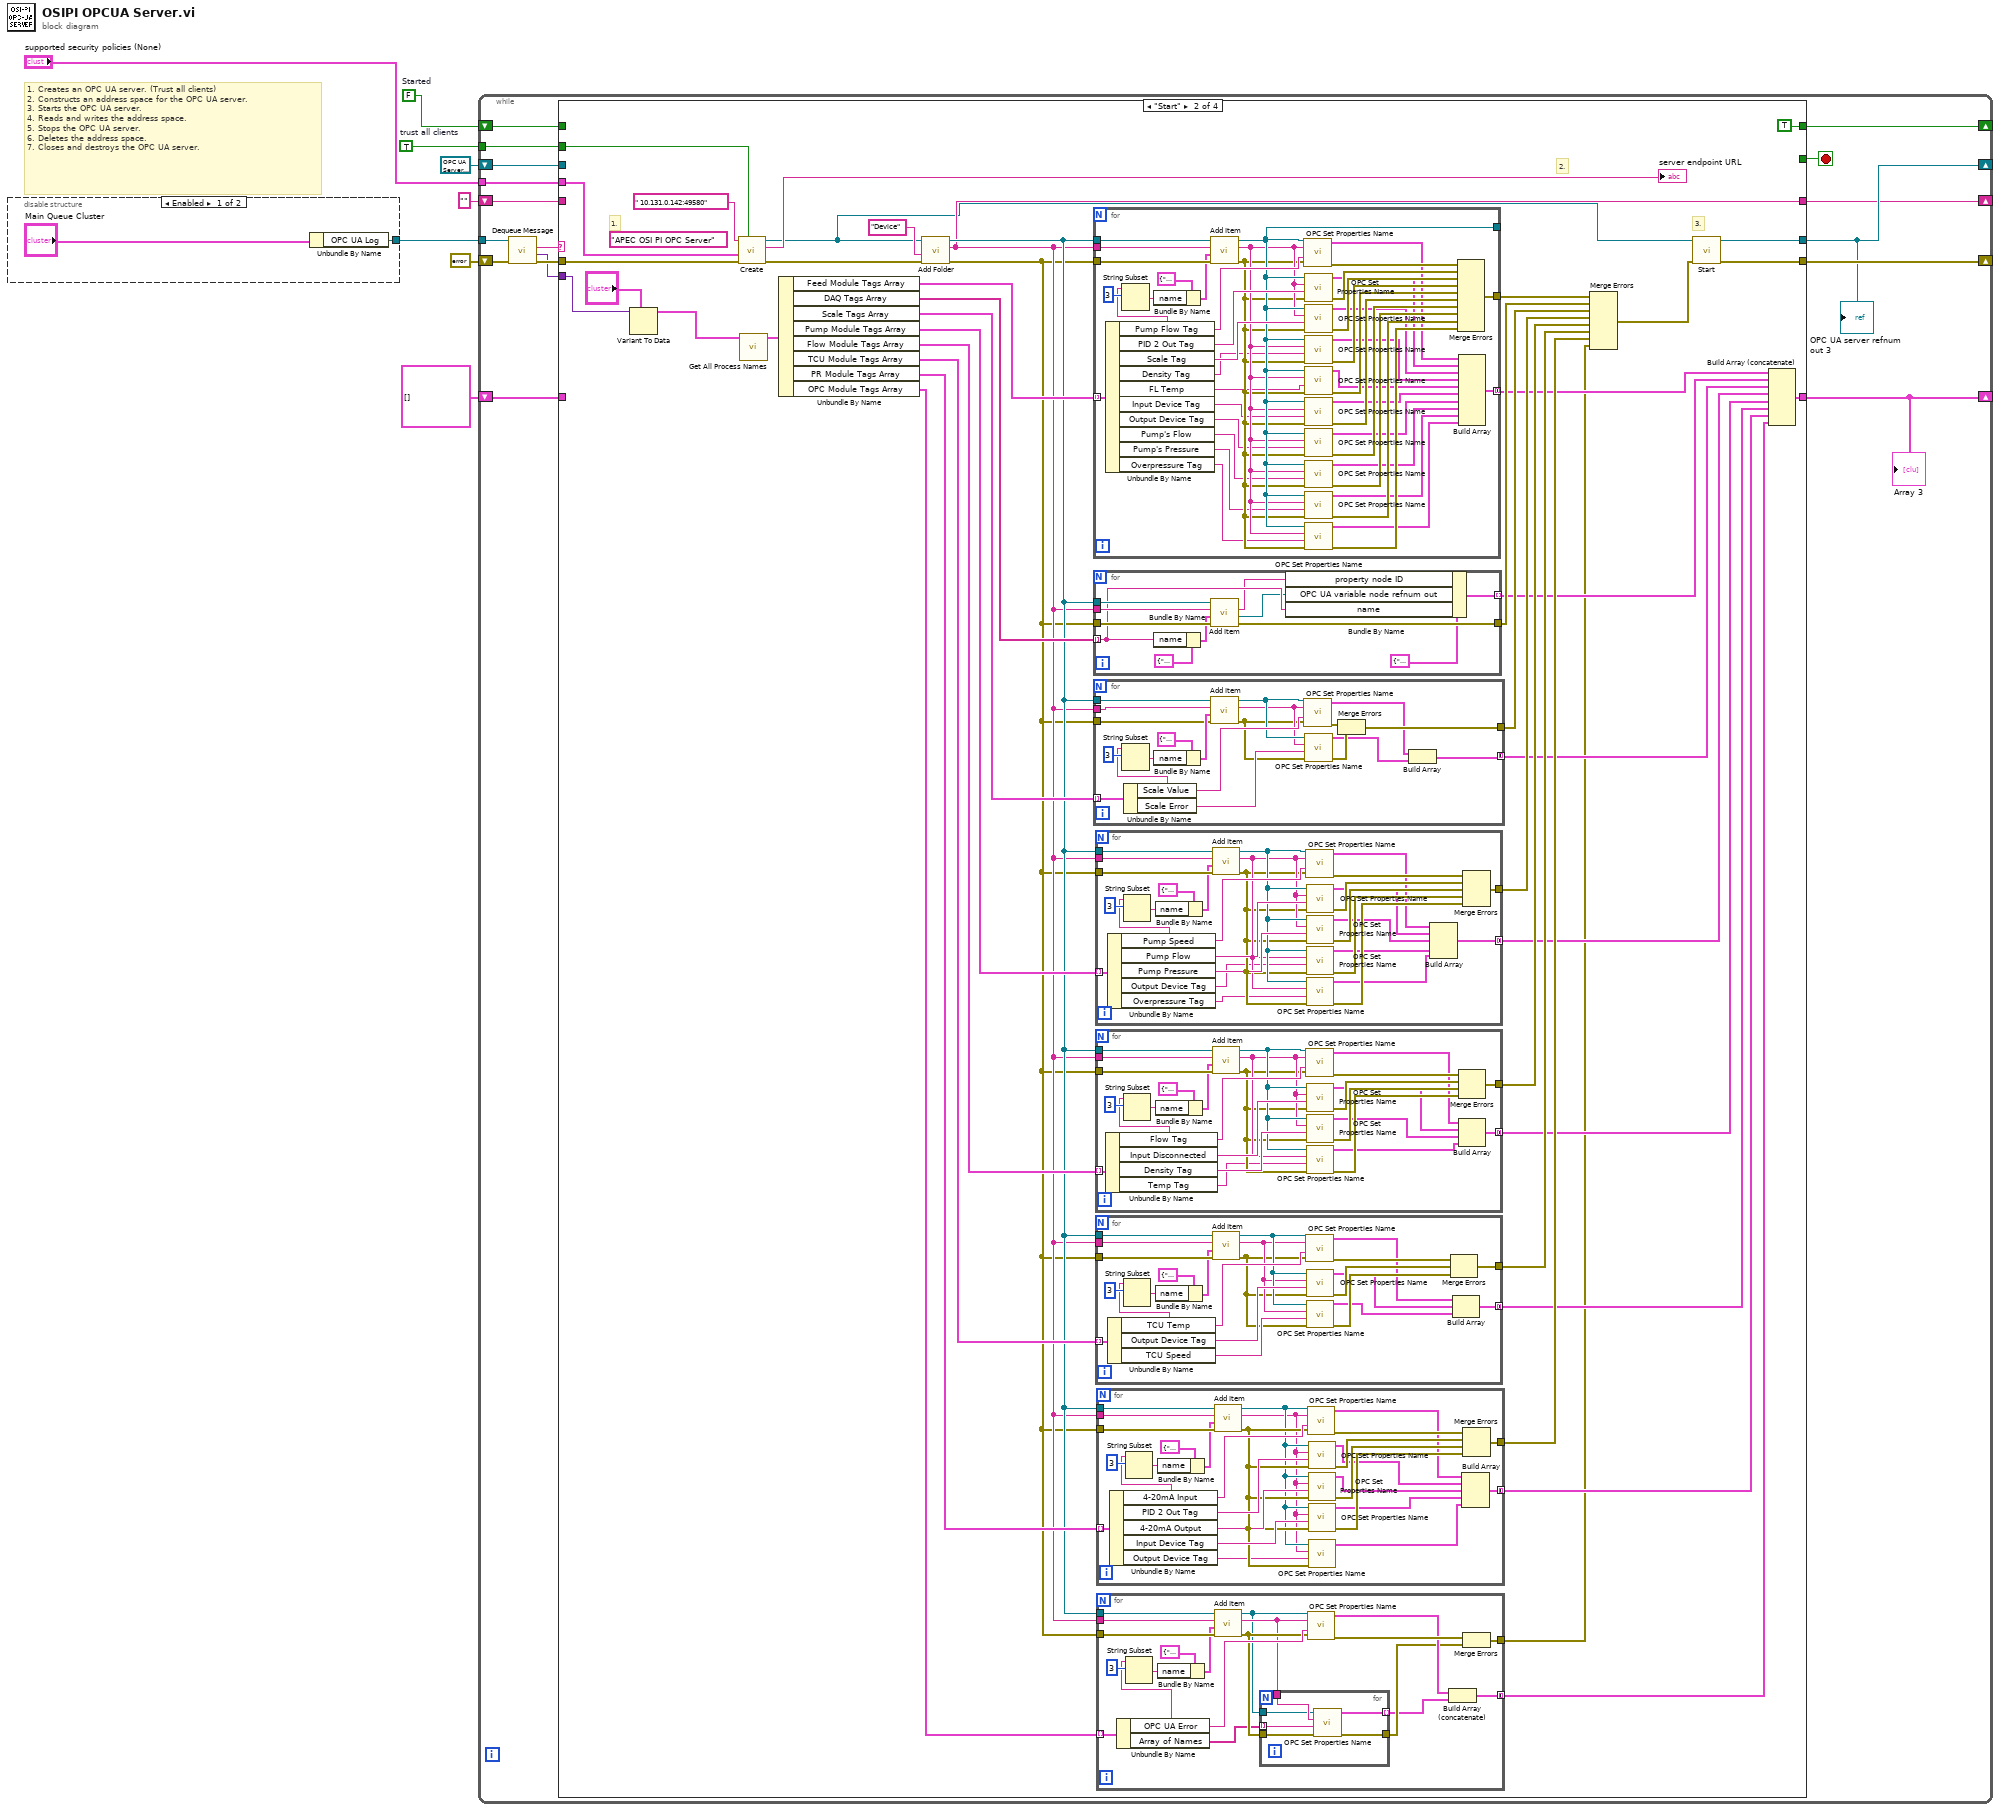
[diagram p0: block diagram]
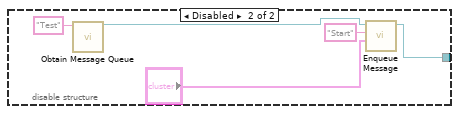
[diagram p2: hidden frame]
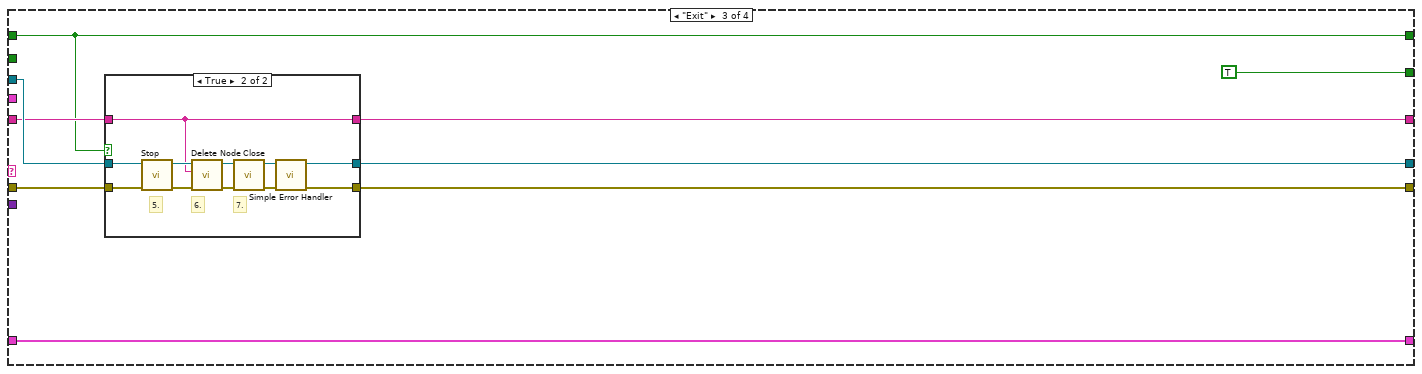
[diagram p4: hidden frame]
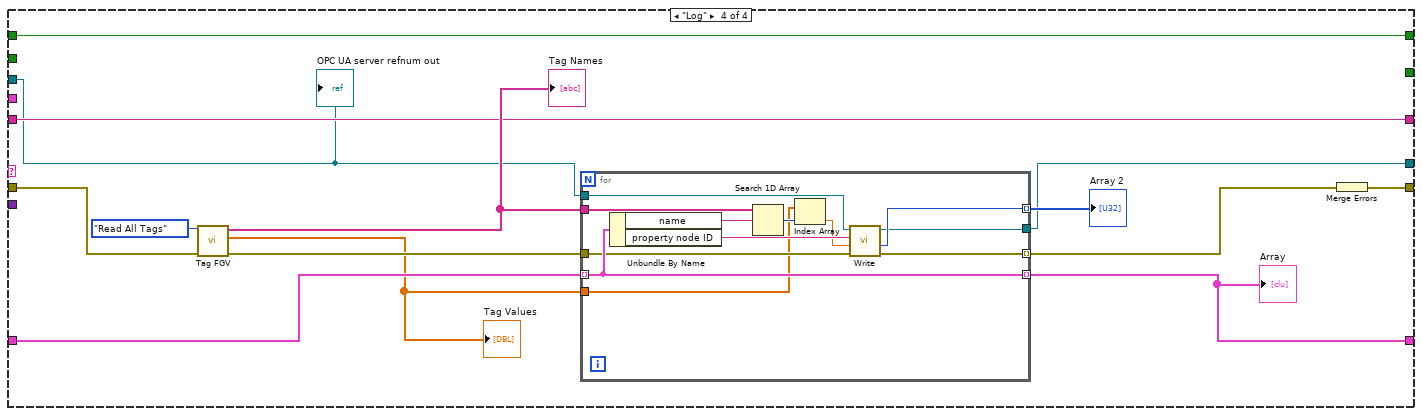
[diagram p6: hidden frame]
diagram:
  w1 = FALSE  # Started
  w8 = TRUE  # trust all clients
  # "1. Creates an OPC UA server. (Trust all clients)\n2. Constructs an address space for the OPC UA server.\n3. Starts the OPC UA server.\n4. Reads and writes the address space.\n5. Stops the OPC UA server.\n6. Deletes the address space.\n7. Closes and destroys the OPC UA server."
  n1 = disable-structure shown="Enabled" {
    disable-tunnel: [w9 w12] -> w6
    frame Enabled {
      n2 = Unbundle By Name("Main Queue Cluster") -> ("OPC UA Log"=w9:refnum<queue>)
    }
    frame Disabled {
      n3 = call "Obtain Message Queue.vi"("name (unnamed)"="Test") -> ("Message Queue"=w11:refnum<queue>)  [unwired: 9 in, 1 out]
      n4 = call-poly "Enqueue Message.vi"("Message Data"="?", "Message"="Start", "Message Queue"=w11) -> ("dup Message Queue"=w12:refnum<queue>)  [unwired: 7 in, 1 out]
    }
  }
  n5 = while {
    tunnel: w6 -> [w31]
    shift-right: [w28] -> _
    shift-left: errorcluster {"status"=FALSE, "code"=0, "source"=""} ("error IO") -> [w27]
    tunnel: w8 -> [w26]
    tunnel: "supported security policies (None)" -> [w25]
    shift-right: [w24] -> _
    shift-left: T4 refnum ("OPC UA server refnum out") -> [w23]
    shift-right: [w22] -> _
    shift-left: T1 "" ("folder node ID") -> [w20]
    shift-right: [w19] -> _
    shift-left: T3 [] -> [w18]
    shift-right: [w17] -> _
    shift-left: w1 -> [w16]
    stop <- w30 stop-if-true
    n6 = call "Dequeue Message.vi"("error in (no error)"=w27, "Message Queue"=w31) -> ("error out"=w29:errorcluster, "Message Data"=w21:variant, "Message"=w32:string)  [unwired: 6 in, 1 out]
    n7 = case shown="\"Start\"" w32 {
      tunnel: [_ _ TRUE _] -> w30
      tunnel: w29 -> [w35 w78 w289 w313]
      tunnel: [w35 w76 w288 w307] -> w28
      tunnel: w26 -> [_ w80 _ _]
      tunnel: w25 -> [_ w79 _ _]
      tunnel: [w36 w77 w286 w304] -> w24
      tunnel: w23 -> [w36 _ w287 w309]
      tunnel: [w37 w43 w282 w314] -> w22
      tunnel: w21 -> [_ w73 _ _]
      tunnel: w20 -> [w37 _ w285 w314]
      tunnel: [w34 w49 w284 w310] -> w19
      tunnel: w18 -> [w34 _ w284 w311]
      tunnel: w16 -> [w33 _ w283 w303]
      tunnel: [w33 TRUE ("Started") w283 w303] -> w17
      frame Default {
      }
      frame "Start" {
        (unwired) "APEC OSI PI OPC Server" ("OPC UA server name")
        # "3."
        # "2."
        # "1."
        n8 = Variant To Data(type="?", Variant=w73) -> (data=w71:T6)  [unwired: 1 in, 1 out]
        n9 = call <vilib>:"Create.vi"("trust all clients (F)"=w80, "error in (no error)"=w78, "supported security policies (None)"=w79, "OPC UA server name"=" 10.131.0.142:49580") -> ("error out"=w75:errorcluster, "server endpoint URL"=→"server endpoint URL":string, "OPC UA server refnum out"=w40:T4)  [unwired: 5 in]
        n10 = call "Get All Process Names.vi"(11:w71) -> ("Module Tags Array Cluster"=w69:T75)  [unwired: 10 in]
        n11 = Unbundle By Name(w69) -> ("Feed Module Tags Array"=w70:T70[], "DAQ Tags Array"=w68:string[], "Scale Tags Array"=w64:T76, "Pump Module Tags Array"=w62:T71[], "Flow Module Tags Array"=w60:T72[], "TCU Module Tags Array"=w58:T73[], "PR Module Tags Array"=w57:T74[], "OPC Module Tags Array"=w41:T77)
        n12 = call <vilib>:"Add Folder.vi"("error in (no error)"=w75, "folder name"="Device", "OPC UA server refnum in"=w40) -> ("error out"=w42:errorcluster, "folder node ID"=w43:T1, "OPC UA server refnum out"=w44:T4)  [unwired: 5 in]
        n13 = for {
          tunnel: w42 -> [w281]
          tunnel: w43 -> [w280]
          tunnel: w44 -> [w279]
          tunnel: [w273] -> w66
          tunnel: [w266] -> _
          tunnel: w70 -> [w276] mode=indexing
          tunnel: [w239] -> w54 mode=concatenating
          n14 = Unbundle By Name(w276) -> ("Pump Flow Tag"=w271:string, "PID 2 Out Tag"=w270:string, "Scale Tag"=w272:string, "Density Tag"=w263:string, "FL Temp"=w262:string, "Input Device Tag"=w261:string, "Output Device Tag"=w260:string, "Pump's Flow"=w259:string, "Pump's Pressure"=w258:string, "Overpressure Tag"=w257:string)
          n15 = String Subset(string=w271, length (rest)=3 ("length (rest)")) -> (substring=w274:string)  [unwired: 1 in]
          n16 = Bundle By Name(cluster=T67 {"name"="Node", "data type"=12, "access level"=3, "description"=""} ("item"), "name"=w274) -> (w277:T67)
          n17 = call <vilib>:"Add Item.vi"("error in (no error)"=w281, "item"=w277, "parent folder node ID"=w280, "OPC UA server refnum in"=w279) -> ("error out"=w264:errorcluster, "item node ID"=w265:T1, "OPC UA server refnum out"=w266:T4)  [unwired: 3 in, 1 out]
          n18 = call "OPC Set Properties Name.vi"("error in (no error)"=w264, "name"=w271, "item node ID"=w265, "Refnum in"=w266) -> ("error out"=w269:errorcluster, "OPC Property cluster"=w249:T68)  [unwired: 6 in]
          n19 = call "OPC Set Properties Name.vi"("error in (no error)"=w264, "name"=w270, "item node ID"=w265, "Refnum in"=w266) -> ("error out"=w268:errorcluster, "OPC Property cluster"=w248:T68)  [unwired: 6 in]
          n20 = call "OPC Set Properties Name.vi"("error in (no error)"=w264, "name"=w272, "item node ID"=w265, "Refnum in"=w266) -> ("error out"=w267:errorcluster, "OPC Property cluster"=w247:T68)  [unwired: 6 in]
          n21 = call "OPC Set Properties Name.vi"("error in (no error)"=w264, "name"=w263, "item node ID"=w265, "Refnum in"=w266) -> ("error out"=w256:errorcluster, "OPC Property cluster"=w246:T68)  [unwired: 6 in]
          n22 = call "OPC Set Properties Name.vi"("error in (no error)"=w264, "name"=w262, "item node ID"=w265, "Refnum in"=w266) -> ("error out"=w255:errorcluster, "OPC Property cluster"=w245:T68)  [unwired: 6 in]
          n23 = call "OPC Set Properties Name.vi"("error in (no error)"=w264, "name"=w261, "item node ID"=w265, "Refnum in"=w266) -> ("error out"=w254:errorcluster, "OPC Property cluster"=w244:T68)  [unwired: 6 in]
          n24 = call "OPC Set Properties Name.vi"("error in (no error)"=w264, "name"=w260, "item node ID"=w265, "Refnum in"=w266) -> ("error out"=w253:errorcluster, "OPC Property cluster"=w243:T68)  [unwired: 6 in]
          n25 = call "OPC Set Properties Name.vi"("error in (no error)"=w264, "name"=w259, "item node ID"=w265, "Refnum in"=w266) -> ("error out"=w252:errorcluster, "OPC Property cluster"=w242:T68)  [unwired: 6 in]
          n26 = call "OPC Set Properties Name.vi"("error in (no error)"=w264, "name"=w258, "item node ID"=w265, "Refnum in"=w266) -> ("error out"=w251:errorcluster, "OPC Property cluster"=w241:T68)  [unwired: 6 in]
          n27 = call "OPC Set Properties Name.vi"("error in (no error)"=w264, "name"=w257, "item node ID"=w265, "Refnum in"=w266) -> ("error out"=w250:errorcluster, "OPC Property cluster"=w240:T68)  [unwired: 6 in]
          n28 = Merge Errors(w269, w268, w267, w256, w255, w254, w253, w252, w251, w250) -> (w273:errorcluster)
          n29 = Build Array(w249, w248, w247, w246, w245, w244, w243, w242, w241, w240) -> (w239:T3)
        }
        n30 = for {
          tunnel: w42 -> [w238]
          tunnel: w43 -> [w237]
          tunnel: w44 -> [w236]
          tunnel: [w233] -> w67
          tunnel: w68 -> [w231] mode=indexing
          tunnel: [w228] -> w53 mode=indexing
          n31 = Bundle By Name(cluster=T67 {"name"="Node", "data type"=11, "access level"=3, "description"=""} ("item"), "name"=w231) -> (w234:T67)
          n32 = call <vilib>:"Add Item.vi"("error in (no error)"=w238, "item"=w234, "parent folder node ID"=w237, "OPC UA server refnum in"=w236) -> ("error out"=w233:errorcluster, "OPC UA variable node refnum out"=w230:T2, "item node ID"=w229:T1)  [unwired: 3 in, 1 out]
          n33 = Bundle By Name(cluster=T68 {"property node ID"="", "OPC UA variable node refnum out"="", "name"=""} ("OPC Property cluster"), "property node ID"=w229, "OPC UA variable node refnum out"=w230, "name"=w231) -> (w228:T68)
        }
        n34 = for {
          tunnel: [w222] -> w63
          tunnel: w64 -> [w225] mode=indexing
          tunnel: w44 -> [w214]
          tunnel: w43 -> [w213]
          tunnel: w42 -> [w212]
          tunnel: [w209] -> w52 mode=concatenating
          n35 = Unbundle By Name(w225) -> ("Scale Value"=w221:string, "Scale Error"=w220:string)
          n36 = String Subset(string=w221, length (rest)=3 ("length (rest)")) -> (substring=w223:string)  [unwired: 1 in]
          n37 = Bundle By Name(cluster=T67 {"name"="Node", "data type"=12, "access level"=3, "description"=""} ("item"), "name"=w223) -> (w226:T67)
          n38 = call <vilib>:"Add Item.vi"("error in (no error)"=w212, "item"=w226, "parent folder node ID"=w213, "OPC UA server refnum in"=w214) -> ("error out"=w215:errorcluster, "item node ID"=w216:T1, "OPC UA server refnum out"=w217:T4)  [unwired: 3 in, 1 out]
          n39 = call "OPC Set Properties Name.vi"("error in (no error)"=w215, "name"=w221, "item node ID"=w216, "Refnum in"=w217) -> ("error out"=w219:errorcluster, "OPC Property cluster"=w211:T68)  [unwired: 6 in]
          n40 = call "OPC Set Properties Name.vi"("error in (no error)"=w215, "name"=w220, "item node ID"=w216, "Refnum in"=w217) -> ("error out"=w218:errorcluster, "OPC Property cluster"=w210:T68)  [unwired: 6 in]
          n41 = Merge Errors(w219, w218) -> (w222:errorcluster)
          n42 = Build Array(w211, w210) -> (w209:T3)
        }
        n43 = for {
          tunnel: w42 -> [w208]
          tunnel: w43 -> [w207]
          tunnel: w44 -> [w206]
          tunnel: [w200] -> w61
          tunnel: w62 -> [w203] mode=indexing
          tunnel: [w181] -> w51 mode=concatenating
          n44 = Unbundle By Name(w203) -> ("Pump Speed"=w198:string, "Pump Flow"=w197:string, "Pump Pressure"=w199:string, "Output Device Tag"=w190:string, "Overpressure Tag"=w189:string)
          n45 = String Subset(string=w198, length (rest)=3 ("length (rest)")) -> (substring=w201:string)  [unwired: 1 in]
          n46 = Bundle By Name(cluster=T67 {"name"="Node", "data type"=12, "access level"=3, "description"=""} ("item"), "name"=w201) -> (w204:T67)
          n47 = call <vilib>:"Add Item.vi"("error in (no error)"=w208, "item"=w204, "parent folder node ID"=w207, "OPC UA server refnum in"=w206) -> ("error out"=w191:errorcluster, "item node ID"=w192:T1, "OPC UA server refnum out"=w193:T4)  [unwired: 3 in, 1 out]
          n48 = call "OPC Set Properties Name.vi"("error in (no error)"=w191, "name"=w198, "item node ID"=w192, "Refnum in"=w193) -> ("error out"=w196:errorcluster, "OPC Property cluster"=w186:T68)  [unwired: 6 in]
          n49 = call "OPC Set Properties Name.vi"("error in (no error)"=w191, "name"=w197, "item node ID"=w192, "Refnum in"=w193) -> ("error out"=w195:errorcluster, "OPC Property cluster"=w185:T68)  [unwired: 6 in]
          n50 = call "OPC Set Properties Name.vi"("error in (no error)"=w191, "name"=w199, "item node ID"=w192, "Refnum in"=w193) -> ("error out"=w194:errorcluster, "OPC Property cluster"=w184:T68)  [unwired: 6 in]
          n51 = call "OPC Set Properties Name.vi"("error in (no error)"=w191, "name"=w190, "item node ID"=w192, "Refnum in"=w193) -> ("error out"=w188:errorcluster, "OPC Property cluster"=w183:T68)  [unwired: 6 in]
          n52 = call "OPC Set Properties Name.vi"("error in (no error)"=w191, "name"=w189, "item node ID"=w192, "Refnum in"=w193) -> ("error out"=w187:errorcluster, "OPC Property cluster"=w182:T68)  [unwired: 6 in]
          n53 = Build Array(w186, w185, w184, w183, w182) -> (w181:T3)
          n54 = Merge Errors(w196, w195, w194, w188, w187) -> (w200:errorcluster)
        }
        n55 = for {
          tunnel: w42 -> [w180]
          tunnel: w43 -> [w179]
          tunnel: w44 -> [w178]
          tunnel: [w172] -> w59
          tunnel: w60 -> [w175] mode=indexing
          tunnel: [w156] -> w50 mode=concatenating
          n56 = Unbundle By Name(w175) -> ("Flow Tag"=w170:string, "Input Disconnected"=w169:string, "Density Tag"=w171:string, "Temp Tag"=w162:string)
          n57 = String Subset(string=w170, length (rest)=3 ("length (rest)")) -> (substring=w173:string)  [unwired: 1 in]
          n58 = Bundle By Name(cluster=T67 {"name"="Node", "data type"=12, "access level"=3, "description"=""} ("item"), "name"=w173) -> (w176:T67)
          n59 = call <vilib>:"Add Item.vi"("error in (no error)"=w180, "item"=w176, "parent folder node ID"=w179, "OPC UA server refnum in"=w178) -> ("error out"=w163:errorcluster, "item node ID"=w164:T1, "OPC UA server refnum out"=w165:T4)  [unwired: 3 in, 1 out]
          n60 = call "OPC Set Properties Name.vi"("error in (no error)"=w163, "name"=w170, "item node ID"=w164, "Refnum in"=w165) -> ("error out"=w168:errorcluster, "OPC Property cluster"=w160:T68)  [unwired: 6 in]
          n61 = call "OPC Set Properties Name.vi"("error in (no error)"=w163, "name"=w169, "item node ID"=w164, "Refnum in"=w165) -> ("error out"=w167:errorcluster, "OPC Property cluster"=w159:T68)  [unwired: 6 in]
          n62 = call "OPC Set Properties Name.vi"("error in (no error)"=w163, "name"=w171, "item node ID"=w164, "Refnum in"=w165) -> ("error out"=w166:errorcluster, "OPC Property cluster"=w158:T68)  [unwired: 6 in]
          n63 = call "OPC Set Properties Name.vi"("error in (no error)"=w163, "name"=w162, "item node ID"=w164, "Refnum in"=w165) -> ("error out"=w161:errorcluster, "OPC Property cluster"=w157:T68)  [unwired: 6 in]
          n64 = Merge Errors(w168, w167, w166, w161) -> (w172:errorcluster)
          n65 = Build Array(w160, w159, w158, w157) -> (w156:T3)
        }
        n66 = for {
          tunnel: w42 -> [w155]
          tunnel: w43 -> [w154]
          tunnel: w44 -> [w153]
          tunnel: [w147] -> w56
          tunnel: w58 -> [w150] mode=indexing
          tunnel: [w134] -> w48 mode=concatenating
          n67 = Unbundle By Name(w150) -> ("TCU Temp"=w145:string, "Output Device Tag"=w144:string, "TCU Speed"=w146:string)
          n68 = String Subset(string=w145, length (rest)=3 ("length (rest)")) -> (substring=w148:string)  [unwired: 1 in]
          n69 = Bundle By Name(cluster=T67 {"name"="Node", "data type"=12, "access level"=3, "description"=""} ("item"), "name"=w148) -> (w151:T67)
          n70 = call <vilib>:"Add Item.vi"("error in (no error)"=w155, "item"=w151, "parent folder node ID"=w154, "OPC UA server refnum in"=w153) -> ("error out"=w138:errorcluster, "item node ID"=w139:T1, "OPC UA server refnum out"=w140:T4)  [unwired: 3 in, 1 out]
          n71 = call "OPC Set Properties Name.vi"("error in (no error)"=w138, "name"=w145, "item node ID"=w139, "Refnum in"=w140) -> ("error out"=w143:errorcluster, "OPC Property cluster"=w137:T68)  [unwired: 6 in]
          n72 = call "OPC Set Properties Name.vi"("error in (no error)"=w138, "name"=w144, "item node ID"=w139, "Refnum in"=w140) -> ("error out"=w142:errorcluster, "OPC Property cluster"=w136:T68)  [unwired: 6 in]
          n73 = call "OPC Set Properties Name.vi"("error in (no error)"=w138, "name"=w146, "item node ID"=w139, "Refnum in"=w140) -> ("error out"=w141:errorcluster, "OPC Property cluster"=w135:T68)  [unwired: 6 in]
          n74 = Merge Errors(w143, w142, w141) -> (w147:errorcluster)
          n75 = Build Array(w137, w136, w135) -> (w134:T3)
        }
        n76 = for {
          tunnel: w42 -> [w133]
          tunnel: w43 -> [w132]
          tunnel: w44 -> [w131]
          tunnel: [w125] -> w55
          tunnel: w57 -> [w128] mode=indexing
          tunnel: [w107] -> w47 mode=concatenating
          n77 = Unbundle By Name(w128) -> ("4-20mA Input"=w123:string, "PID 2 Out Tag"=w122:string, "4-20mA Output"=w124:string, "Input Device Tag"=w117:string, "Output Device Tag"=w113:string)
          n78 = String Subset(string=w123, length (rest)=3 ("length (rest)")) -> (substring=w126:string)  [unwired: 1 in]
          n79 = Bundle By Name(cluster=T67 {"name"="Node", "data type"=12, "access level"=3, "description"=""} ("item"), "name"=w126) -> (w129:T67)
          n80 = call <vilib>:"Add Item.vi"("error in (no error)"=w133, "item"=w129, "parent folder node ID"=w132, "OPC UA server refnum in"=w131) -> ("error out"=w116:errorcluster, "item node ID"=w114:T1, "OPC UA server refnum out"=w115:T4)  [unwired: 3 in, 1 out]
          n81 = call "OPC Set Properties Name.vi"("error in (no error)"=w116, "name"=w123, "item node ID"=w114, "Refnum in"=w115) -> ("error out"=w121:errorcluster, "OPC Property cluster"=w112:T68)  [unwired: 6 in]
          n82 = call "OPC Set Properties Name.vi"("error in (no error)"=w116, "name"=w122, "item node ID"=w114, "Refnum in"=w115) -> ("error out"=w120:errorcluster, "OPC Property cluster"=w111:T68)  [unwired: 6 in]
          n83 = call "OPC Set Properties Name.vi"("error in (no error)"=w116, "name"=w124, "item node ID"=w114, "Refnum in"=w115) -> ("error out"=w119:errorcluster, "OPC Property cluster"=w110:T68)  [unwired: 6 in]
          n84 = call "OPC Set Properties Name.vi"("error in (no error)"=w116, "name"=w117, "item node ID"=w114, "Refnum in"=w115) -> ("error out"=w118:errorcluster, "OPC Property cluster"=w109:T68)  [unwired: 6 in]
          n85 = call "OPC Set Properties Name.vi"("error in (no error)"=w116, "name"=w113, "item node ID"=w114, "Refnum in"=w115) -> ("OPC Property cluster"=w108:T68)  [unwired: 6 in, 1 out]
          n86 = Build Array(w112, w111, w110, w109, w108) -> (w107:T3)
          n87 = Merge Errors(w121, w120, w119, w118) -> (w125:errorcluster)
        }
        n88 = for {
          tunnel: w42 -> [w100]
          tunnel: w43 -> [w99]
          tunnel: w44 -> [w98]
          tunnel: [w92] -> w45
          tunnel: w41 -> [w95] mode=indexing
          tunnel: [w88] -> w46 mode=concatenating
          n89 = Unbundle By Name(w95) -> ("OPC UA Error"=w91:string, "Array of Names"=w83:string[])
          n90 = String Subset(string=w91, length (rest)=3 ("length (rest)")) -> (substring=w93:string)  [unwired: 1 in]
          n91 = Bundle By Name(cluster=T67 {"name"="Node", "data type"=12, "access level"=3, "description"=""} ("item"), "name"=w93) -> (w96:T67)
          n92 = call <vilib>:"Add Item.vi"("error in (no error)"=w100, "item"=w96, "parent folder node ID"=w99, "OPC UA server refnum in"=w98) -> ("error out"=w87:errorcluster, "item node ID"=w86:T1, "OPC UA server refnum out"=w85:T4)  [unwired: 3 in, 1 out]
          n93 = for {
            tunnel: w87 -> [w106]
            tunnel: w86 -> [w105]
            tunnel: w85 -> [w104]
            tunnel: [w103] -> w84
            tunnel: w83 -> [w102] mode=indexing
            tunnel: [w101] -> w82 mode=indexing
            n94 = call "OPC Set Properties Name.vi"("error in (no error)"=w106, "name"=w102, "item node ID"=w105, "Refnum in"=w104) -> ("error out"=w103:errorcluster, "OPC Property cluster"=w101:T68)  [unwired: 6 in]
          }
          n95 = call "OPC Set Properties Name.vi"("error in (no error)"=w87, "name"=w91, "item node ID"=w86, "Refnum in"=w85) -> ("error out"=w90:errorcluster, "OPC Property cluster"=w89:T68)  [unwired: 6 in]
          n96 = Build Array (concatenate)(w89, w82) -> (w88:T3)
          n97 = Merge Errors(w90, w84) -> (w92:errorcluster)
        }
        n98 = Merge Errors(w66, w67, w63, w61, w59, w56, w55, w45) -> (w65:errorcluster)
        n99 = call <vilib>:"Start.vi"("error in (no error)"=w65, "OPC UA server refnum in"=w40) -> ("error out"=w76:errorcluster, "OPC UA server refnum out"=w77:T4)  [unwired: 7 in, 1 out]
        n100 = Build Array (concatenate)(w54, w53, w52, w51, w50, w48, w47, w46) -> (w49:T3)
      }
      frame "Exit" {
        n101 = case shown="True" w283 {
          tunnel: w289 -> [w292 w298]
          tunnel: [w292 w297] -> w288
          tunnel: w287 -> [w293 w296]
          tunnel: [w293 w295] -> w286
          tunnel: w285 -> [w291 w294]
          tunnel: [w291 w294] -> w282
          frame False {
          }
          frame True {
            # "7."
            # "6."
            # "5."
            n102 = call <vilib>:"Stop.vi"("error in (no error)"=w298, "OPC UA server refnum in"=w296) -> ("error out"=w300:errorcluster, "OPC UA server refnum out"=w301:T4)  [unwired: 8 in]
            n103 = call <vilib>:"Delete Node.vi"("error in (no error)"=w300, "node ID"=w294, "OPC UA server refnum in"=w301) -> ("error out"=w302:errorcluster, "OPC UA server refnum out"=w295:T4)  [unwired: 7 in]
            n104 = call <vilib>:"Close.vi"("error in (no error)"=w302, "OPC UA server refnum in"=w295) -> ("error out"=w299:errorcluster)  [unwired: 9 in]
            n105 = call <vilib>:"Simple Error Handler.vi"("error in (no error)"=w299) -> ("error out"=w297:errorcluster)  [unwired: 4 in, 4 out]
          }
        }
      }
      frame "Log" {
        n106 = call "Tag FGV.vi"("error in (no error)"=w313, "Operation"=Tag_FGV_Operation_Enum."Read All Tags") -> ("error out"=w312:errorcluster, "Tag Values"=w306:dbl[], "Tag Names"=w315:string[])  [unwired: 4 in, 3 out]
        "Tag Values" <- w306
        "Tag Names" <- w315
        n107 = for {
          tunnel: w315 -> [w327]
          tunnel: w312 -> [w322]
          tunnel: w311 -> [w328] mode=indexing
          tunnel: [w328] -> w310 mode=indexing
          tunnel: w309 -> [w323]
          tunnel: [w321] -> w308 mode=indexing
          tunnel: w306 -> [w320]
          tunnel: [w318] -> w305 mode=indexing
          tunnel: [w317] -> w304
          n108 = Unbundle By Name(w328) -> ("name"=w326:string, "property node ID"=w324:T1)
          n109 = Search 1D Array(1D array=w327, element=w326) -> (index of element=w325:i32)  [unwired: 1 in]
          n110 = Index Array(array=w320, index=w325) -> (element=w319:dbl)
          n111 = call-poly <vilib>:"Write.vi"("error in (no error)"=w322, "value"=w319, "node ID"=w324, "OPC UA server refnum in"=w323) -> ("error out"=w321:errorcluster, "status"=w318:T5, "OPC UA server refnum out"=w317:T4)  [unwired: 5 in]
        }
        "Array" <- w310
        "Array 2" <- w305
        n112 = Merge Errors(w308) -> (w307:errorcluster)
        "OPC UA server refnum out" <- w309
      }
    }
    "OPC UA server refnum out 3" <- w24
    "Array 3" <- w19
  }
